vi "AndorAcqSingleImgToIMAQ.vi"(4 "Maximum":sgl, 6 "Minimum":sgl, 7 "Image Name":string, 8 "error in (no error)":errorcluster, 9 "Exposure Time":dbl, 10 "Image Area Width":i32, 11 "Image Area Height":i32) -> (0 "error out":errorcluster, 3 "Image Dst Out":T1)   [LabVIEW 2018, in "AndorOWN.lvlib"]
uses:
  AndorOWN.lvlib
  <vilib>/vision/Image Controls.llb/IMAQ Image.ctl
  Andor SDK/AndorSDK.lvlib
  <vilib>/vision/NI_Vision_Development_Module.lvlib
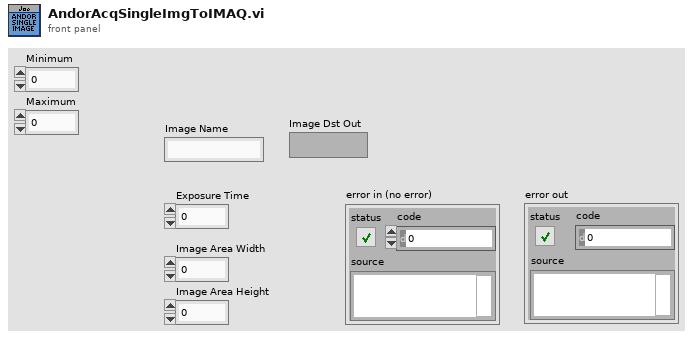
[diagram p1: front panel]
types:
  T1 = typedef "IMAQ Image.ctl" = refnum<image>
  T2 = enum32{"Linear", "Log", "Exp", "Square", "Square root", "Power X", "Power 1/X"}
  T3 = typedef "Image Type" = u32
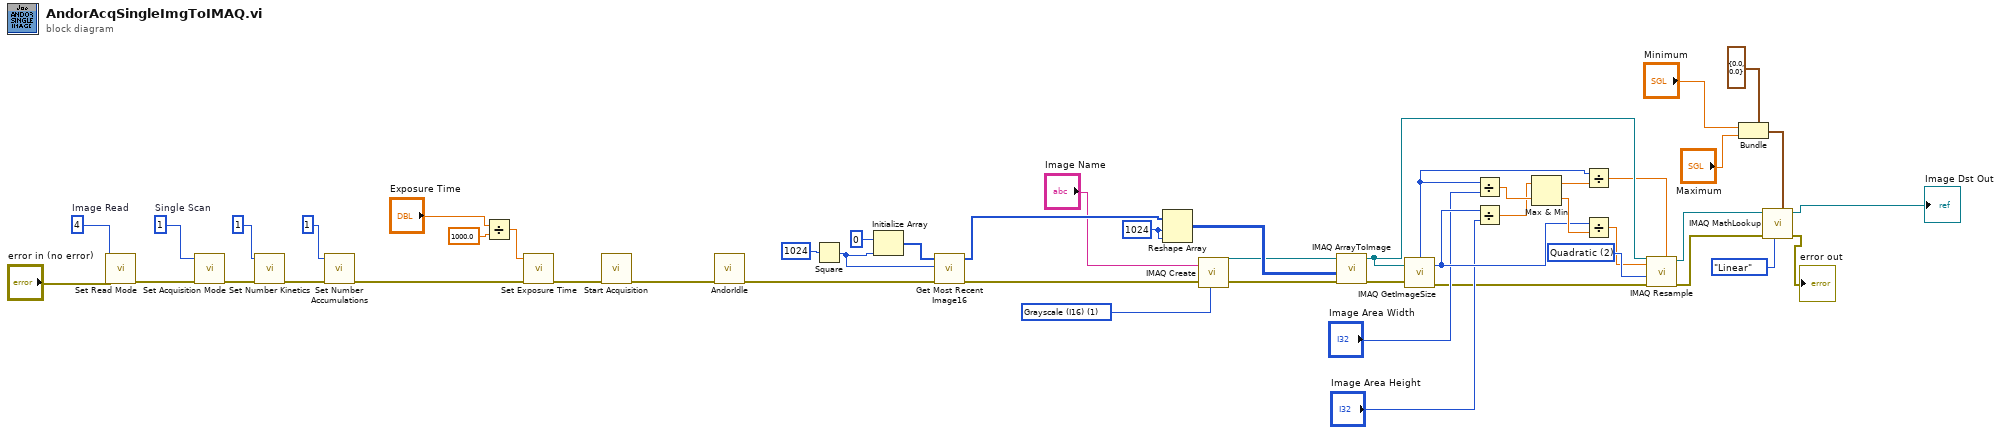
[diagram p0: block diagram]
diagram:
  w25 = u32 2 items=["Zero Order", "Bi-Linear", "Quadratic", "Cubic Spline"] ("Interpolation Type")
  w24 = T3 1 items=["Grayscale (U8)", "Grayscale (I16)", "Grayscale (SGL)", "Complex (CSG)", "RGB (U32)", "HSL (U32)", "RGB (U64)", "Grayscale (U16)"] ("Image Type")
  w23 = 1024 ("dimension size")
  w39 = 1  # Single Scan
  w40 = 4  # Image Read
  n1 = call "Set Read Mode.vi"("error in (no error)"="error in (no error)", "mode"=w40) -> ("error out"=w46:errorcluster)  [unwired: 8 in, 1 out]
  n2 = call "Set Acquisition Mode.vi"("error in (no error)"=w46, "mode"=w39) -> ("error out"=w47:errorcluster)  [unwired: 8 in, 1 out]
  n3 = call "Set Number Kinetics.vi"("error in (no error)"=w47, "number"=1) -> ("error out"=w48:errorcluster)  [unwired: 8 in, 1 out]
  n4 = call "Set Number Accumulations.vi"("error in (no error)"=w48, "number"=1) -> ("error out"=w49:errorcluster)  [unwired: 8 in, 1 out]
  n5 = Divide(x="Exposure Time", y=sgl 1000.0) -> (x/y=w36:dbl)
  n6 = call "Set Exposure Time.vi"("error in (no error)"=w49, "time"=w36) -> ("error out"=w45:errorcluster)  [unwired: 8 in, 1 out]
  n7 = call "Start Acquisition.vi"("error in (no error)"=w45) -> ("error out"=w44:errorcluster)  [unwired: 9 in, 1 out]
  n8 = call "AndorIdle.vi"("error in (no error)"=w44) -> ("error out"=w43:errorcluster)  [unwired: 9 in, 1 out]
  n9 = Square(x=1024) -> (x^2=w30:i32)
  n10 = Initialize Array(i16 0 ("element"), w30) -> (w31:i16[])
  n11 = call "Get Most Recent Image16.vi"("error in (no error)"=w43, "size"=w30, "arr"=w31) -> ("error out"=w42:errorcluster, "arr out"=w50:i16[])  [unwired: 6 in, 1 out]
  n12 = Reshape Array(w50, w23, w23) -> (w27:i16[][])
  n13 = call "IMAQ Create"("Image Name"="Image Name", "Image Type"=w24, "error in (no error)"=w42) -> ("New Image"=w26:T1, "error out"=w12:errorcluster)  [unwired: 2 in]
  n14 = call "IMAQ ArrayToImage"("error in (no error)"=w12, "Image Pixels (I16)"=w27, "Image"=w26) -> ("error out"=w11:errorcluster, "Image Out"=w22:T1)  [unwired: 7 in]
  n15 = call "IMAQ GetImageSize"("Image"=w22, "error in (no error)"=w11) -> ("Y Resolution"=w16:i32, "X Resolution"=w19:i32, "error out"=w10:errorcluster)  [unwired: 2 in]
  n16 = Divide(x=w19, y="Image Area Width") -> (x/y=w29:dbl)
  n17 = Divide(x=w16, y="Image Area Height") -> (x/y=w28:dbl)
  n18 = Max & Min(x=w28, y=w29) -> (max(x,y)=w21:dbl, min(x,y)=w17:dbl)
  n19 = Divide(x=w19, y=w21) -> (x/y=w20:dbl)
  n20 = Divide(x=w16, y=w17) -> (x/y=w18:dbl)
  n21 = call "IMAQ Resample"("X Resolution"=w20, "Y Resolution"=w18, "error in (no error)"=w10, "Interpolation Type"=w25, "Image Src"=w22) -> ("error out"=w5:errorcluster, "Image Dst Out"=w6:T1)  [unwired: 5 in]
  n22 = Bundle(cluster=cluster{"Minimum":sgl, "Maximum":sgl} {"Minimum"=0.0, "Maximum"=0.0} ("Range"), "Minimum"="Minimum", "Maximum"="Maximum") -> (w7:cluster{"Minimum":sgl, "Maximum":sgl})
  n23 = call "IMAQ MathLookup"("Range"=w7, "Operator"=T2."Linear", "error in (no error)"=w5, "Image Src"=w6) -> ("error out"=→"error out":errorcluster, "Image Dst Out"=→"Image Dst Out":T1)  [unwired: 6 in]
